vi "FilterDTOFromNative.vi"(8 "error in (no error)":errorcluster, 11 "Filter":T1={"mode"=enum."Mirror", "levelMin"=enum."INFO", "levelMax"=enum."INFO", "tagPrefix"=""}) -> (0 "error out":errorcluster, 3 "FilterDTO":T4={"mode"="Mirror", "levelMin"="INFO", "levelMax"="INFO", "tagPrefix"=""})   [LabVIEW 2026, in "Lumberjack.lvlib"]
uses:
  Lumberjack.lvlib
  TypeDefs/ConfigDTO/FilterDTO.ctl
  TypeDefs/Filter.ctl
  TypeDefs/FilterMode.ctl
  TypeDefs/Severity.ctl
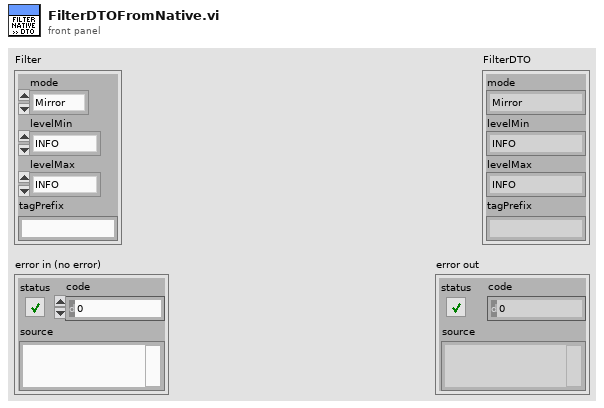
[diagram p1: front panel]
types:
  T1 = typedef "Lumberjack.lvlib/Filter.ctl" = cluster{"mode":T2, "levelMin":T3, "levelMax":T3, "tagPrefix":string}
  T2 = typedef "Lumberjack.lvlib/FilterMode.ctl" = enum16{"Mirror", "Routed"}
  T3 = typedef "Lumberjack.lvlib/Severity.ctl" = enum16{"OFF", "FATAL", "ERROR", "WARN", "INFO", "DEBUG", "TRACE", "ALL"}
  T4 = typedef "Lumberjack.lvlib/FilterDTO.ctl" = cluster{"mode":string, "levelMin":string, "levelMax":string, "tagPrefix":string}
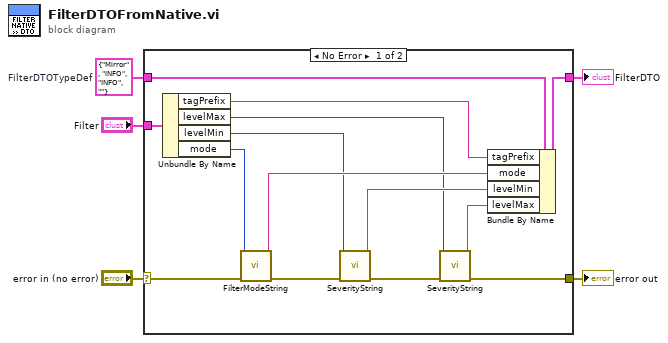
[diagram p0: block diagram]
diagram:
  w1 = T4 {"mode"="Mirror", "levelMin"="INFO", "levelMax"="INFO", "tagPrefix"=""}  # FilterDTOTypeDef
  n1 = case shown="No Error" "error in (no error)" {
    selector: "error in (no error)" -> [w19 w21]
    tunnel: [w16 w21] -> w3
    tunnel: "Filter" -> [w14 _]
    tunnel: w1 -> [w12 w20]
    tunnel: [w15 w20] -> w2
    frame No Error {
      n2 = Unbundle By Name(w14) -> ("tagPrefix"=w13:string, "levelMax"=w7:T3, "levelMin"=w9:T3, "mode"=w11:T2)
      n3 = call "FilterModeString.vi"("error in (no error)"=w19, "FilterMode"=w11) -> ("error out"=w18:errorcluster, "FilterModeString"=w10:string)  [unwired: 8 in]
      n4 = call "SeverityString.vi"("error in (no error)"=w18, "Severity"=w9) -> ("error out"=w17:errorcluster, "SeverityString"=w8:string)  [unwired: 8 in]
      n5 = call "SeverityString.vi"("error in (no error)"=w17, "Severity"=w7) -> ("error out"=w16:errorcluster, "SeverityString"=w6:string)  [unwired: 8 in]
      n6 = Bundle By Name(cluster=w12, "tagPrefix"=w13, "mode"=w10, "levelMin"=w8, "levelMax"=w6) -> (w15:T4)
    }
    frame Error {
    }
  }
  "FilterDTO" <- w2
  "error out" <- w3
